vi "LIA 5783 Getting Started.vi"() -> ()   [LabVIEW 2017]
uses:
  <vilib>/userdefined/Silver/nirio_resource_slv.ctl
  Program Files (x86)/National Instruments/LabVIEW 2017/examples/FlexRIO/IO Modules/NI 5783/NI 5783 - Getting Started/Controls/Clock Select.ctl
  <vilib>/Analysis/4window.llb/windowTd.ctl
  <vilib>/measure/maspectr.llb/Power Spectrum and PSD Export Mode.ctl
  <vilib>/FPGAPlugInAG/PXIe-7976R/niLvFpga_Open_PXIe-7976R.vi
  <vilib>/rvi/interface/common/dynamic/niFpgaDynamicAddResources.vi
  <vilib>/rvi/interface/common/niFpgaWaitOnOcc.vi
  <vilib>/Utility/error.llb/Error Cluster From Error Code.vi
  <vilib>/rvi/errors/niLvFpgaAdjustHostInterfaceError.vi
  <instrlib>/_niInstr/Streaming/v1/Host/Public/Start Finite Stream.vi
  <instrlib>/_niInstr/Streaming/v1/Host/Public/Wait for Stream.vi
  <vilib>/measure/maspectr.llb/FFT Power Spectrum and PSD for 1 Chan.vi
  <instrlib>/_niInstr/Streaming/v1/Host/Public/Start Continuous Stream.vi
  <vilib>/FPGAPlugInAG/Dynamic/niLvFpga_Close_Dynamic.vi
  <vilib>/rvi/interface/nirviOpenFPGA/nirviOpenFPGA.xnode
  Program Files (x86)/National Instruments/LabVIEW 2017/examples/FlexRIO/IO Modules/NI 5783/NI 5783 - Getting Started/FPGA Bitfiles/NI 5783 - Getting Started_7976R.lvbitx
  <vilib>/rvi/interface/nirviMethod/nirviMethod.xnode
  <vilib>/rvi/interface/nirviReadWriteControl/nirviReadWriteControl.xnode
  <vilib>/rvi/interface/nirviCloseFPGA/nirviCloseFPGA.xnode
  <vilib>/rvi/errors/niLvFpgaMergeErrorWithErrorCode.vi
  <vilib>/rvi/interface/Simulation/niFpgaSimulationCallBeginRW.vi
  <instrlib>/_niInstr/Streaming/v1/Host/niInstr Streaming v1 Host.lvlib
  NiFpgaLv.dll
  <vilib>/FPGAPlugInAG/Dynamic/niLvFpga_ConfigureFifo_Dynamic.vi
  <vilib>/FPGAPlugInAG/Dynamic/niLvFpga_StartFifo_Dynamic.vi
  <vilib>/FPGAPlugInAG/Dynamic/niLvFpga_WriteFifo_Dynamic.vi
  <vilib>/FPGAPlugInAG/Dynamic/niLvFpga_ReadFifo_Dynamic.vi
  <vilib>/Analysis/NI_AALPro.lvlib
  <vilib>/measure/NI_MAPro.lvlib
panel:
  out "mean":dbl
  out "Numeric":dbl
  out "size(s)":i32
  in  "averaging parameters":T1={"averaging mode"=enum."RMS averaging", "weighting mode"=enum."Exponential", "number of averages"=10} {"number of averages" min=1}
  in  "restart averaging (F)":bool
  out "Power Spectrum (dBm)":cluster{"f0":dbl, "df":dbl, "magnitude":dbl[]}[](graph)
  in  "Trigger Type":enum8{"Immediate", "Data Trigger", "TRIG input"}(ring)
  in  "Clock Select":T2 items=["Internal Clock", "Internal Clock w/ Ref via CLK/REF IN", "Internal Clock w/ Ref via Sync Clock", "External Clock via CLK/REF IN"]
  in  "Rate of External Sample Clock (MHz)":u16=100 min=60 max=100 step=1
  in  "AO Channel":T3(ring)
  in  "Data Trigger When":enum8{"Trigger Above", "Trigger Below"}(ring)
  in  "Sampling Info":cluster{"Fs":dbl, "#s":dbl}={"Fs"=200000000.0, "#s"=1000.0} {"Fs" format="%#_6p"}
  in  "Update Waveform":bool
  in  "Signal Type":T4(ring)
  in  "Frequency (Hz)":dbl=1000000.0 format="%0.2p"
  in  "Amplitude (V)":dbl=0.25 format="%0.2p"
  out "AO":waveform(dbl)(graph)
  out "AI":waveform(dbl)[](graph)
  out "Error Out":errorcluster
  in  "Data Trigger Level (V)":dbl
  in  "stop":bool
  in  "Record Size":u16=8192
  in  "RIO Resource":T5="RIO0"
  # "Resource Configuration"
  # "AI Configuration"
  # "Ignored when Internal Clock is selected"
  # "AI Configuration"
  # "A0 Configuration"
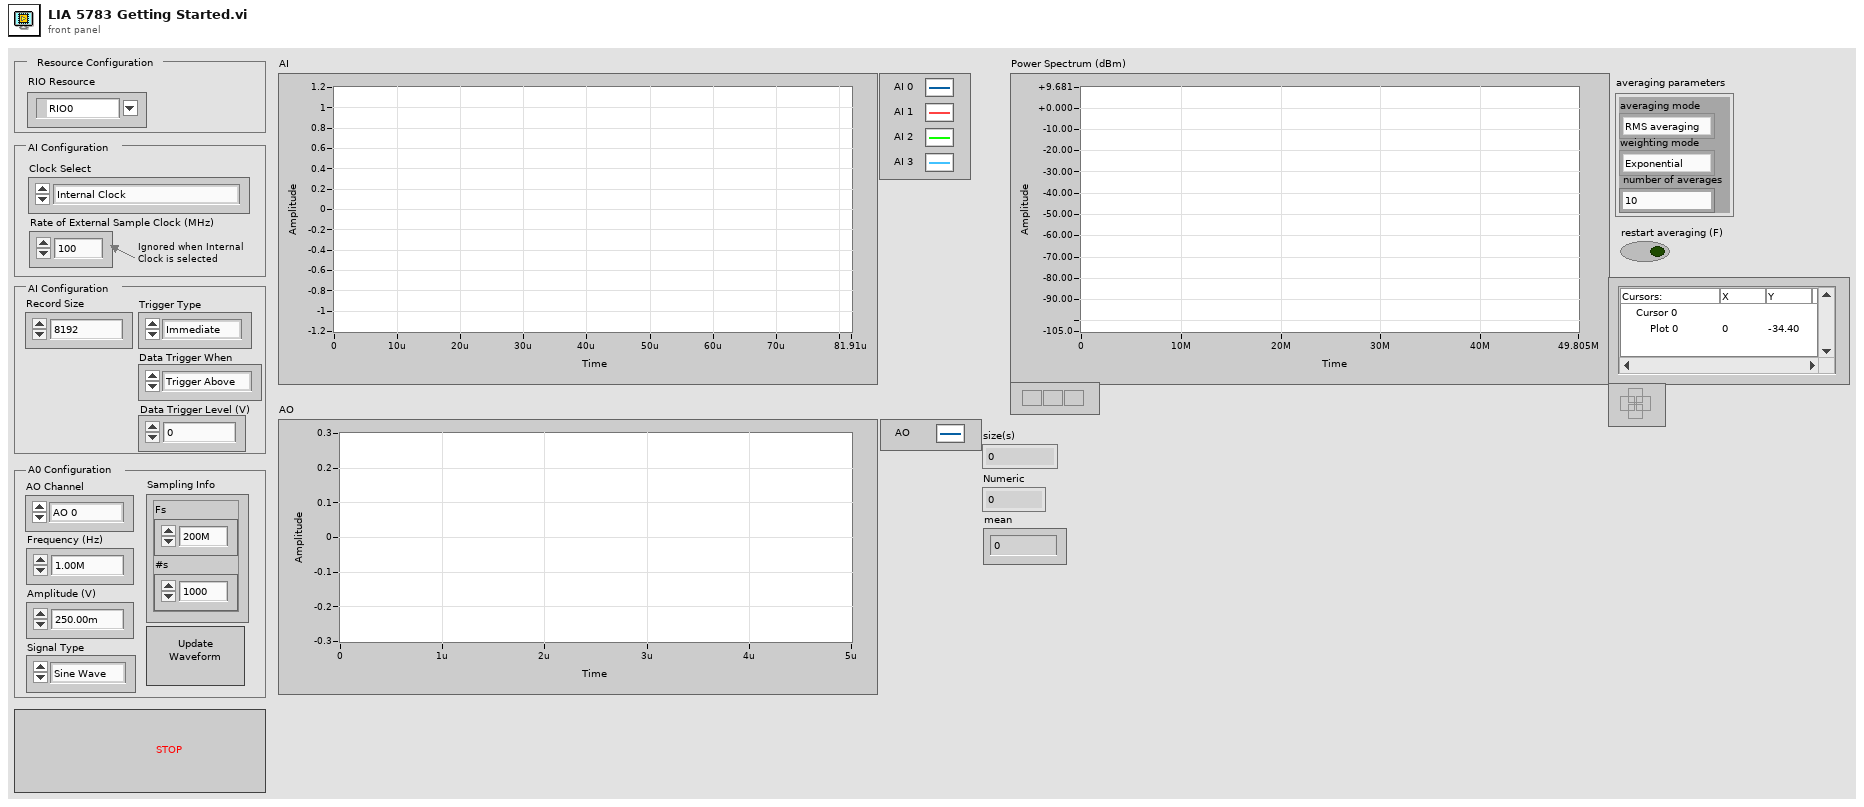
[diagram p1: front panel]
types:
  T1 = cluster{"averaging mode":enum16{"No averaging", "Vector averaging", "RMS averaging", "Peak hold"}, "weighting mode":enum16{"Linear", "Exponential"}, "number of averages":u32}
  T2 = typedef "Clock Select.ctl" = u16
  T3 = enum8{"AO 0", "AO 1", "AO 2", "AO 3", "AO 0, AO 1, AO 2, AO 3", "None"}
  T4 = enum16{"Sine Wave", "Triangle Wave", "Square Wave", "Sawtooth Wave"}
  T5 = typedef "nirio_resource_slv.ctl" = tag
  T6 = cluster{"level":i16, "trigger when":enum8{"Trigger Above", "Trigger Below"}}
  T7 = typedef "NI_AALPro.lvlib/windowTd.ctl" = u32
  T8 = typedef "NI_MAPro.lvlib/Power Spectrum and PSD Export Mode.ctl" = u16
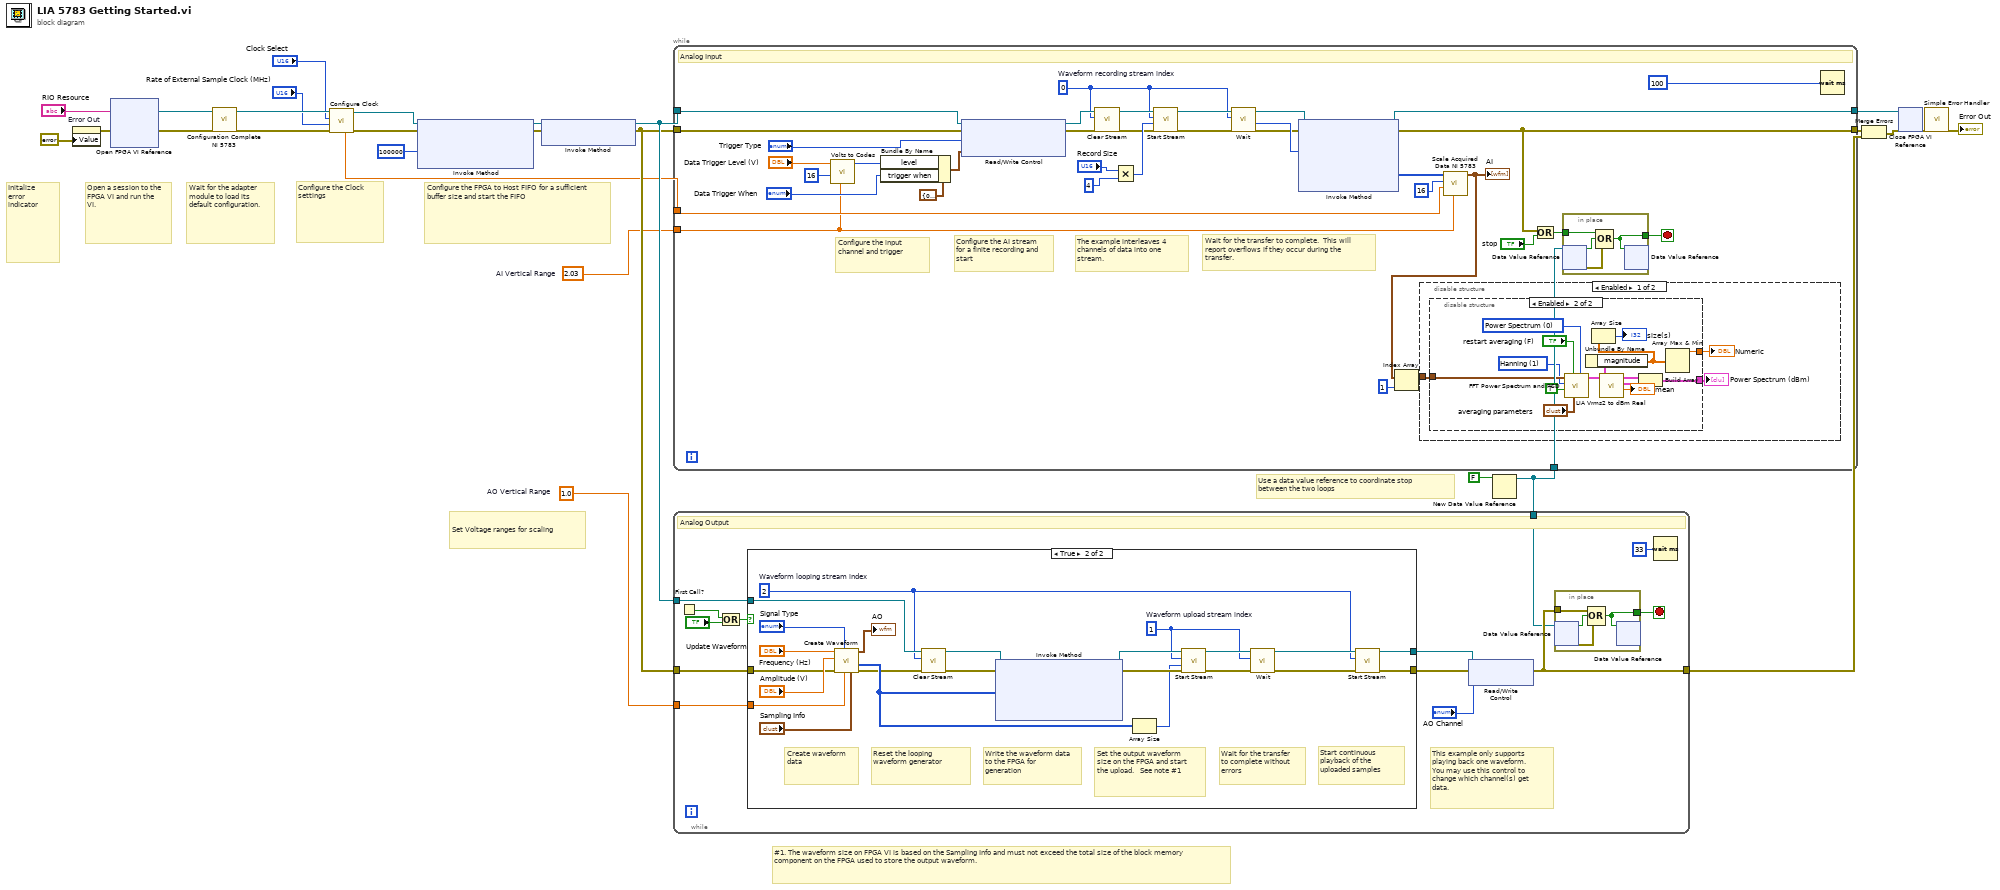
[diagram p0: block diagram]
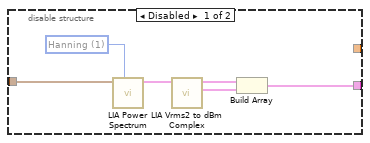
[diagram p3: hidden frame]
diagram:
  w11 = 2.03  # AI Vertical Range
  w10 = 1.0  # AO Vertical Range
  # "Configure the Clock settings"
  # "Configure the FPGA to Host FIFO for a sufficient buffer size and start the FIFO"
  # "Wait for the adapter module to load its default configuration."
  # "Open a session to the FPGA VI and run the VI."
  # "Use a data value reference to coordinate stop between the two loops"
  # "Set Voltage ranges for scaling"
  # "Initalize error indicator"
  # "#1. The waveform size on FPGA VI is based on the Sampling Info and must not exceed the total size of the block memory component on the FPGA used to store the output waveform."
  n1 = property on="Error Out" class="Clust (strict)"("Value"=errorcluster {"status"=FALSE, "code"=0, "source"=""} ("error out")) -> (error out=w21:errorcluster)  [unwired: 2 in, 1 out]
  n2 = xnode "Open FPGA VI Reference"("error in"=w21, "resource name"="RIO Resource") -> ("FPGA VI Reference Out"=w9:refnum<k20>, "error out"=w8:errorcluster)
  n3 = call "Configuration Complete NI 5783.vi"("error in"=w8, "FPGA VI Reference In"=w9) -> ("error out"=w6:errorcluster, "FPGA VI Reference Out"=w7:refnum<k20>)  [unwired: 7 in, 1 out]
  n4 = call "Configure Clock.vi"("error in (no error)"=w6, "Rate of External Sample Clock (MHz)"="Rate of External Sample Clock (MHz)", "Clock Select"="Clock Select", "FPGA VI Reference In"=w7) -> ("error out"=w4:errorcluster, "FPGA VI Reference Out"=w5:refnum<k20>, "Sampling Rate"=w1:dbl)  [unwired: 3 in, 2 out]
  n5 = xnode "Invoke Method"("FPGA VI Reference In"=w5, "error in"=w4, "Requested Depth"=u32 100000) -> ("FPGA VI Reference Out"=w15:refnum<k20>, "error out"=w14:errorcluster)  [unwired: 1 out]
  n6 = xnode "Invoke Method"("FPGA VI Reference In"=w15, "error in"=w14) -> ("FPGA VI Reference Out"=w19:refnum<k20>, "error out"=w16:errorcluster)
  n7 = New Data Value Reference(data value=FALSE ("Stopped")) -> (data value reference=w17:refnum<data-value>)  [unwired: 1 in, 1 out]
  n8 = while {
    tunnel: w16 -> [w40]
    tunnel: [w33] -> w24
    tunnel: w19 -> [w39]
    tunnel: w10 -> [w36]
    tunnel: w17 -> [w32]
    stop <- w31 stop-if-true
    # "This example only supports playing back one waveform.  You may use this control to change which channel(s) get data."
    # "Analog Output"
    n9 = First Call?() -> (First Call?: T/F=w29:bool)
    n10 = Or(x=w29, y="Update Waveform") -> (x .or. y?=w30:bool)
    n11 = case shown="True" w30 {
      tunnel: w40 -> [w45 w48]
      tunnel: [w46 w59] -> w35
      tunnel: [w45 w58] -> w34
      tunnel: w39 -> [w46 w52]
      tunnel: w36 -> [_ w64]
      frame False {
      }
      frame True {
        w50 = 2  # Waveform looping stream index
        w53 = 1  # Waveform upload stream index
        # "Reset the looping waveform generator"
        # "Start continuous playback of the uploaded samples"
        # "Wait for the transfer to complete without errors"
        # "Set the output waveform size on the FPGA and start the upload.   See note #1"
        # "Write the waveform data to the FPGA for generation"
        # "Create waveform data"
        n12 = call "Create Waveform.vi"("sampling info"="Sampling Info", "range (Vpp)"=w64, "signal type"="Signal Type", "error in (no error)"=w48, "amplitude"="Amplitude (V)", "frequency"="Frequency (Hz)") -> ("error out"=w47:errorcluster, "Waveform Data"=w61:i16[], "Output Waveform (V)"=→"AO":waveform(dbl))  [unwired: 2 in, 1 out]
        n13 = call <instrlib>:"Clear Stream.vi"("error in (no error)"=w47, "stream index"=w50, "refnum in"=w52) -> ("error out"=w49:errorcluster, "refnum out"=w51:refnum<k20>)  [unwired: 7 in]
        n14 = xnode "Invoke Method"("FPGA VI Reference In"=w51, "error in"=w49, "Data"=w61) -> ("FPGA VI Reference Out"=w63:refnum<k20>, "error out"=w62:errorcluster)  [unwired: 1 in, 1 out]
        n15 = Array Size(array=w61) -> (size(s)=w60:i32)
        n16 = call-poly <instrlib>:"Start Stream.vi"("error in (no error)"=w62, "num samples"=w60, "stream index"=w53, "refnum in"=w63) -> ("error out"=w56:errorcluster, "refnum out"=w57:refnum<k20>)  [unwired: 6 in]
        n17 = call-poly <instrlib>:"Wait.vi"("error in (no error)"=w56, "stream index"=w53, "refnum in"=w57) -> ("error out"=w54:errorcluster, "refnum out"=w55:refnum<k20>)  [unwired: 5 in, 2 out]
        n18 = call-poly <instrlib>:"Start Stream.vi"("error in (no error)"=w54, "stream index"=w50, "refnum in"=w55) -> ("error out"=w58:errorcluster, "refnum out"=w59:refnum<k20>)  [unwired: 7 in]
      }
    }
    n19 = xnode "Read/Write Control"("FPGA VI Reference In"=w35, "error in"=w34, "AO Channel"="AO Channel") -> ("error out"=w33:errorcluster)  [unwired: 1 out]
    n20 = in-place {
      in-place-border: [w42] -> w31
      in-place-border: w33 -> [w44]
      n21 = in-place-dvr #1(w32) -> (w43:bool, w41:errorcluster)
      n22 = Compound Arithmetic op=OR(w44, w43, w41) -> (w42:bool)
      n23 = in-place-dvr #1(w42) -> ()  [unwired: 2 out]
    }
    n24 = Wait (ms)(milliseconds to wait=u32 33) -> ()  [unwired: 1 out]
  }
  n25 = while {
    tunnel: [w104] -> w27
    tunnel: w19 -> [w103]
    tunnel: w11 -> [w82]
    tunnel: w17 -> [w100]
    tunnel: w16 -> [w102]
    tunnel: [w88] -> w26
    tunnel: w1 -> [w83]
    stop <- w101 stop-if-true
    w73 = 0  # Waveform recording stream index
    # "The example interleaves 4 channels of data into one stream."
    # "Wait for the transfer to complete.  This will report overflows if they occur during the transfer."
    # "Configure the AI stream for a finite recording and start"
    # "Configure the input channel and trigger"
    # "Analog Input"
    n26 = call "Volts to Codes.vi"("range (Vpp)"=w82, "Number of Bits"=i16 16, "Volts In"="Data Trigger Level (V)") -> ("ADC Codes Out"=w84:i16)  [unwired: 8 in]
    n27 = Bundle By Name(cluster=T6 {"level"=0, "trigger when"=enum."Trigger Above"} ("Trigger Configuration"), "level"=w84, "trigger when"="Data Trigger When") -> (w87:T6)
    n28 = xnode "Read/Write Control"("FPGA VI Reference In"=w103, "error in"=w102, "Trigger Type"="Trigger Type", "Trigger Configuration"=w87) -> ("FPGA VI Reference Out"=w77:refnum<k20>, "error out"=w76:errorcluster)
    n29 = call <instrlib>:"Clear Stream.vi"("error in (no error)"=w76, "stream index"=w73, "refnum in"=w77) -> ("error out"=w75:errorcluster, "refnum out"=w74:refnum<k20>)  [unwired: 7 in]
    n30 = Multiply(x="Record Size", y=u16 4) -> (x*y=w79:u16)
    n31 = call-poly <instrlib>:"Start Stream.vi"("error in (no error)"=w75, "num samples"=w79, "stream index"=w73, "refnum in"=w74) -> ("error out"=w93:errorcluster, "refnum out"=w91:refnum<k20>)  [unwired: 6 in]
    n32 = call-poly <instrlib>:"Wait.vi"("error in (no error)"=w93, "stream index"=w73, "refnum in"=w91) -> ("error out"=w89:errorcluster, "samples transferred"=w92:u64, "refnum out"=w90:refnum<k20>)  [unwired: 5 in, 1 out]
    n33 = xnode "Invoke Method"("FPGA VI Reference In"=w90, "error in"=w89, "Number of Elements"=w92) -> ("FPGA VI Reference Out"=w104:refnum<k20>, "error out"=w88:errorcluster, "Data"=w96:i16[])  [unwired: 1 in, 1 out]
    n34 = call "Scale Acquired Data NI 5783.vi"("range (V)"=w82, "Sample Rate"=w83, "Number of Bits"=i16 16, "Data In"=w96) -> ("Data"=w72:waveform(dbl)[])  [unwired: 7 in]
    "AI" <- w72
    n35 = Index Array(array=w72, index=1) -> (element=w71:waveform(dbl))
    n36 = disable-structure shown="Enabled" {
      disable-tunnel: w71 -> [w107 _]
      frame Enabled {
        n37 = disable-structure shown="Enabled" {
          disable-tunnel: [w109 w122] -> w108
          disable-tunnel: w107 -> [w113 w128]
          disable-tunnel: [_ w117] -> w106
          frame Disabled {
            w114 = T7 1 items=["Rectangle"=0, "Hanning"=1, "Hamming"=2, "Blackman-Harris"=3, "Exact Blackman"=4, "Blackman"=5, "Flat Top"=6, "4 Term B-Harris "=7, "7 Term B-Harris"=8, "Low Sidelobe"=9, "Blackman Nuttall"=11, "Triangle"=30, "Bartlett-Hanning"=31, "Bohman"=32, "Parzen"=33, "Welch"=34, "Kaiser"=60, "Dolph-Chebyshev"=61, "Gaussian"=62] ("window")
            n38 = call "LIA Power Spectrum.vi"("window"=w114, "waveform"=w113) -> ("Waveform Graph 5"=w112:cluster{"x0":dbl, "dx":dbl, "Y":dbl[]})  [unwired: 9 in]
            n39 = call "LIA Vrms2 to dBm Complex.vi"("Power Spectrum / PSD"=w112) -> ("output cluster"=w110:cluster{"f0":dbl, "df":dbl, "magnitude":dbl[]}, "Power Spectrum / PSD (dBm)"=w111:cluster{"f0":dbl, "df":dbl, "magnitude":dbl[]})  [unwired: 9 in]
            n40 = Build Array(w111, w110) -> (w109:cluster{"f0":dbl, "df":dbl, "magnitude":dbl[]}[])
          }
          frame Enabled {
            w123 = T8 0 items=["Power Spectrum", "Power Spectral Density"] ("export mode")
            w126 = T7 1 items=["Rectangle"=0, "Hanning"=1, "Hamming"=2, "Blackman-Harris"=3, "Exact Blackman"=4, "Blackman"=5, "Flat Top"=6, "4 Term B-Harris "=7, "7 Term B-Harris"=8, "Low Sidelobe"=9, "Blackman Nuttall"=11, "Triangle"=30, "Bartlett-Hanning"=31, "Bohman"=32, "Parzen"=33, "Welch"=34, "Kaiser"=60, "Dolph-Chebyshev"=61, "Gaussian"=62] ("window")
            n41 = call-poly <vilib>:"FFT Power Spectrum and PSD.vi"("export mode"=w123, "averaging parameters"="averaging parameters", "restart averaging (F)"="restart averaging (F)", "dB On (F)"=TRUE, "window"=w126, "time signal"=w128) -> ("Power Spectrum / PSD"=w120:cluster{"f0":dbl, "df":dbl, "magnitude":dbl[]})  [unwired: 2 in, 3 out]
            n42 = call "LIA Vrms2 to dBm Real.vi"("Power Spectrum / PSD"=w120) -> ("mean"=→"mean":dbl, "output cluster"=w121:cluster{"f0":dbl, "df":dbl, "magnitude":dbl[]}, "Power Spectrum / PSD (dBm)"=w115:cluster{"f0":dbl, "df":dbl, "magnitude":dbl[]})  [unwired: 8 in]
            n43 = Unbundle By Name(w115) -> ("magnitude"=w118:dbl[])
            n44 = Array Size(array=w118) -> (size(s)=→"size(s)":i32)
            n45 = Build Array(w115, w121) -> (w122:cluster{"f0":dbl, "df":dbl, "magnitude":dbl[]}[])
            n46 = Array Max & Min(array=w118) -> (max value=w117:dbl)  [unwired: 3 out]
          }
        }
        "Power Spectrum (dBm)" <- w108
        "Numeric" <- w106
      }
      frame Disabled {
      }
    }
    n47 = Or(x=w88, y="stop") -> (x .or. y?=w99:bool)
    n48 = in-place {
      in-place-border: [w130] -> w101
      in-place-border: w99 -> [w132]
      n49 = in-place-dvr #2(w100) -> (w131:bool, w129:errorcluster)
      n50 = Compound Arithmetic op=OR(w132, w131, w129) -> (w130:bool)
      n51 = in-place-dvr #2(w130) -> ()  [unwired: 2 out]
    }
    n52 = Wait (ms)(milliseconds to wait=u32 100) -> ()  [unwired: 1 out]
  }
  n53 = Merge Errors(w26, w24) -> (w25:errorcluster)
  n54 = xnode "Close FPGA VI Reference"("FPGA VI Reference In"=w27, "error in"=w25) -> ("error out"=w23:errorcluster)
  n55 = call <vilib>:"Simple Error Handler.vi"("error in (no error)"=w23) -> ("error out"=→"Error Out":errorcluster)  [unwired: 4 in, 4 out]
